vi "mask_off_ROIs.vi"(8 "Error In":errorcluster, 9 "ROIs In":T1(array[cluster]), 10 "Image Name":string, 11 "Path":path) -> (0 "Error Out":errorcluster, 3 "ROIs out":T1(array[cluster]))   [LabVIEW 2019]
uses:
  mask_off_rois_states_enum_typedef.ctl
panel:
  in  "Done":bool
  out "Image":T2(plugin-control)
  # "Mask ROIs"
  # "Using a closed form tool (circle, rectangle, etc) select\na region for which you wish to KEEP any ROIs (i.e. an\narea of valid grains). Click done when this is complete."
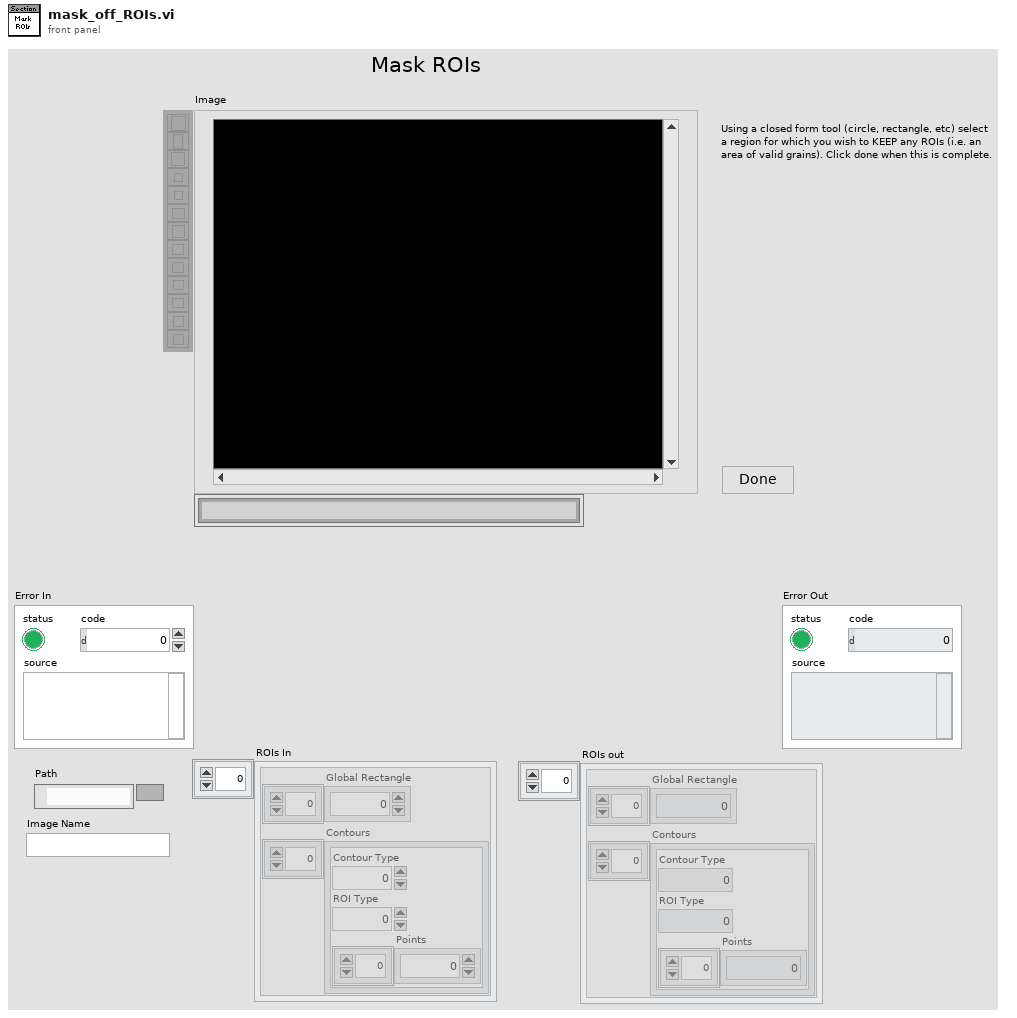
[diagram p1: front panel]
types:
  T1 = cluster{"Global Rectangle":i32[], "Contours":cluster{"Contour Type":u32, "ROI Type":u32, "Points":i32[]}[]}[]
  T2 = typedef "IMAQ Image.ctl" = refnum<image>
  T3 = typedef "mask_off_rois_states_enum_typedef.ctl" = enum16{"Shutdown", "Wait", "Initialize"}
  T4 = cluster{"Global Rectangle":i32[], "Contours":cluster{"Contour Type":u32, "ROI Type":u32, "Points":i32[]}[]}
  T5 = typedef "ROI Descriptor" = cluster{"Global Rectangle":i32[], "Contours":cluster{"ID":enum32{"External", "Internal"}, "Type":u32, "Coordinates":i32[]}[]}
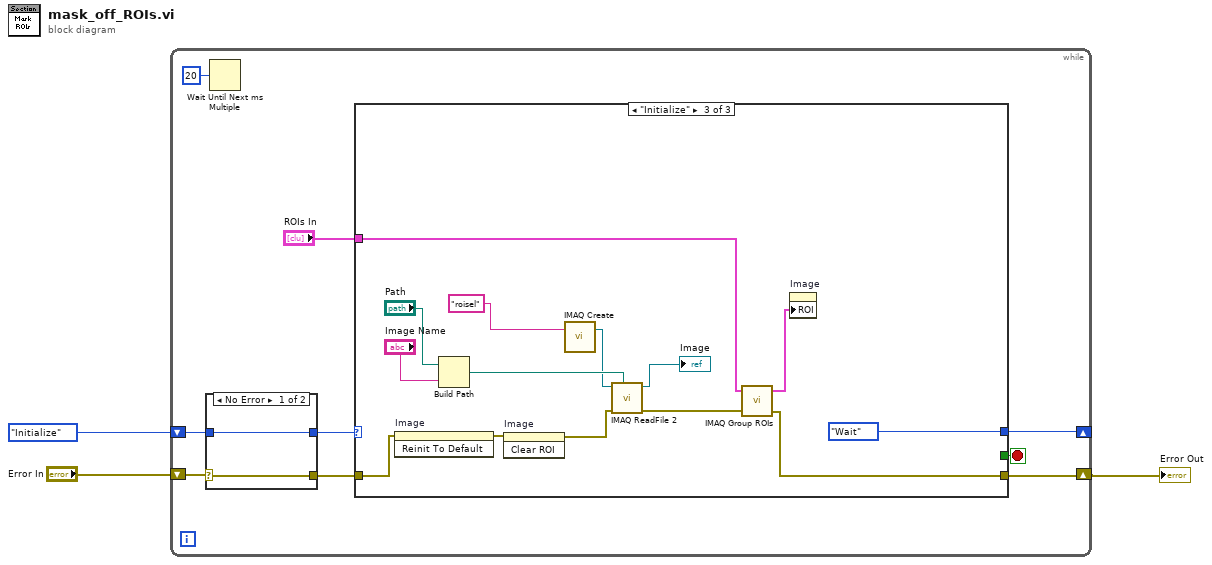
[diagram p0: block diagram]
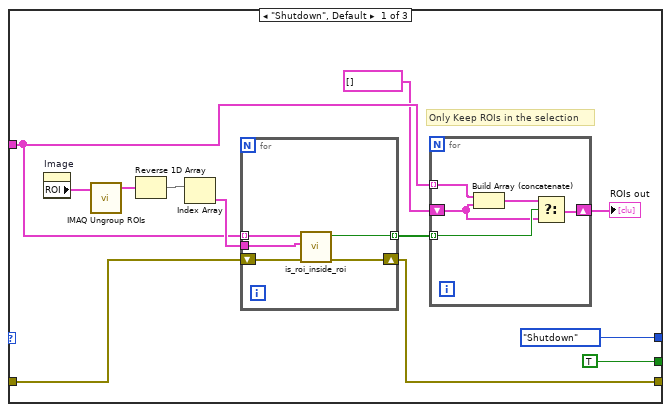
[diagram p2: hidden frame]
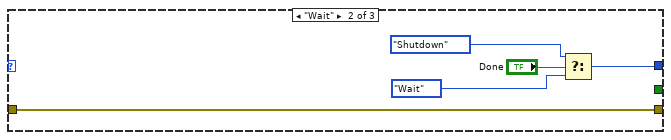
[diagram p3: hidden frame]
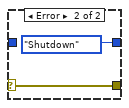
[diagram p4: hidden frame]
diagram:
  n1 = while {
    shift-right: [w7] -> _
    shift-left: mask_off_rois_states_enum_typedef."Initialize" -> [w11]
    shift-right: [w6] -> w1
    shift-left: "Error In" -> [w12]
    stop <- w4 stop-if-true
    n2 = case shown="No Error" w12 {
      selector: w12 -> [w54 w56]
      tunnel: [w55 mask_off_rois_states_enum_typedef."Shutdown"] -> w9
      tunnel: w11 -> [w55 _]
      tunnel: [w54 w56] -> w8
      frame No Error {
      }
      frame Error {
      }
    }
    n3 = Wait Until Next ms Multiple(millisecond multiple=u32 20) -> ()  [unwired: 1 out]
    n4 = case shown="\"Initialize\"" w9 {
      tunnel: w8 -> [w22 w35 w42]
      tunnel: [mask_off_rois_states_enum_typedef."Shutdown" w38 mask_off_rois_states_enum_typedef."Wait"] -> w7
      tunnel: [w13 w35 w44] -> w6
      tunnel: "ROIs In" -> [w17 _ w43]
      tunnel: [TRUE _ _] -> w4
      frame "Shutdown", Default {
        # "Only Keep ROIs in the selection"
        n5 = property on="Image" class="ImageControl"() -> ("ROI"=w21:T4)  [unwired: 2 in, 2 out]
        n6 = call "IMAQ Ungroup ROIs"("ROI Descriptor"=w21) -> ("ROI Descriptors out"=w20:T5[])  [unwired: 3 in, 1 out]
        n7 = Reverse 1D Array(array=w20) -> (reversed array=w19:T5[])
        n8 = Index Array(array=w19) -> (element=w18:T5)  [unwired: 1 in]
        n9 = for {
          shift-right: [w30] -> w13
          shift-left: w22 -> [w34]
          tunnel: w17 -> [w33] mode=indexing
          tunnel: w18 -> [w32]
          tunnel: [w31] -> w16 mode=indexing
          n10 = call "is_roi_inside_roi.vi"("Error In"=w34, "ROI Outer"=w32, "ROI Inner"=w33) -> ("Error Out"=w30:errorcluster, "Inner is inside Outer"=w31:bool)  [unwired: 7 in]
        }
        n11 = for {
          tunnel: w17 -> [w27] mode=indexing
          tunnel: w16 -> [w28] mode=indexing
          shift-right: [w29] -> w14
          shift-left: T1 [] ("Array") -> [w25]
          n12 = Build Array (concatenate)(w27, w25) -> (w26:T1)
          n13 = Select(t=w26, s=w28, f=w25) -> (s? t:f=w29:T1)
        }
        "ROIs out" <- w14
      }
      frame "Wait" {
        n14 = Select(t=mask_off_rois_states_enum_typedef."Shutdown", s="Done", f=mask_off_rois_states_enum_typedef."Wait") -> (s? t:f=w38:T3)
      }
      frame "Initialize" {
        n15 = invoke on="Image" class="ImageControl" method="Reinit To Default"(error in=w42) -> (error out=w41:errorcluster)  [unwired: 2 in, 2 out]
        n16 = Build Path(base path="Path", name or relative path="Image Name") -> (appended path=w50:path)
        n17 = invoke on="Image" class="ImageControl" method="Clear ROI"(error in=w41) -> (error out=w40:errorcluster)  [unwired: 2 in, 2 out]
        n18 = call "IMAQ Create"("Image Name"="roisel") -> ("New Image"=w49:T2)  [unwired: 4 in, 1 out]
        n19 = call "IMAQ ReadFile 2"("File Path"=w50, "error in (no error)"=w40, "Image"=w49) -> ("error out"=w45:errorcluster, "Image Out"=→"Image":T2)  [unwired: 4 in, 3 out]
        n20 = call "IMAQ Group ROIs"("error in (no error)"=w45, "ROI Descriptors"=w43) -> ("error out"=w44:errorcluster, "ROI Descriptor out"=w47:T5)  [unwired: 2 in]
        n21 = property on="Image" class="ImageControl"("ROI"=w47) -> ()  [unwired: 2 in, 2 out]
      }
    }
  }
  "Error Out" <- w1
